vi "RCM Filter String MHLC.vi"(8 "error in (no error)":errorcluster, 10 "Data":variant, 11 "Message Log in":refnum<class "Message Log.lvclass">) -> (0 "error out":errorcluster, 3 "Message Log out":refnum<class "Message Log.lvclass">)   [LabVIEW 2017, in "Message Log.lvclass"]
doc: "Filter string on selected column"
uses:
  Message Log.lvclass
  rql_RCM Filter String.ctl
  Listbox Selection.ctl
  <vilib>/Utility/miscctls.llb/LVRowAndColumnTypeDef.ctl
  Message Log.lvclass/Message Log.ctl
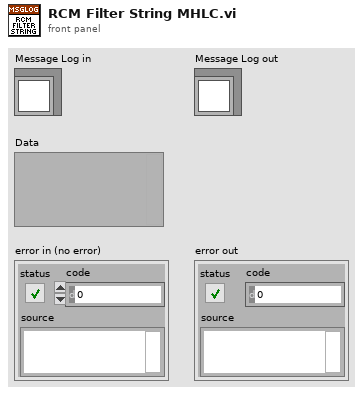
[diagram p1: front panel]
types:
  T1 = typedef "Message Log.lvclass/rql_RCM Filter String.ctl" = cluster{"RCM Listbox Data":T2}
  T2 = typedef "Message Log.lvclass/Listbox Selection.ctl" = cluster{"Cell Position":T3, "Row":string[]}
  T3 = typedef "LVRowAndColumnTypeDef.ctl" = cluster{"Row":i32, "Column":i32}
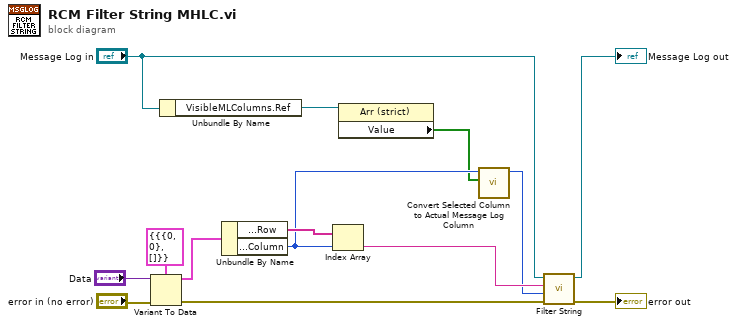
[diagram p0: block diagram]
diagram:
  n1 = Variant To Data(error in="error in (no error)", type=T1 {"RCM Listbox Data"={"Cell Position"={"Row"=0, "Column"=0}, "Row"=[]}} ("Data"), Variant="Data") -> (data=w13:T1, error out=w4:errorcluster)
  n2 = Unbundle By Name("Message Log in") -> ("VisibleMLColumns.Ref"=w8:refnum<vi>)
  n3 = Unbundle By Name(w13) -> ("RCM Listbox Data.Row"=w10:string[], "RCM Listbox Data.Cell Position.Column"=w9:i32)
  n4 = Index Array(array=w10, index=w9) -> (element=w6:string)
  n5 = property class="Arr (strict)"(reference=w8) -> ("Value"=w7:bool[])  [unwired: 1 in, 2 out]
  n6 = call "Convert Selected Column to Actual Message Log Column.vi"("Visible ML Columns"=w7, "Selected Column"=w9) -> ("Actual Column"=w5:i32)  [unwired: 9 in]
  n7 = call "Filter String.vi"("error in (no error)"=w4, "Actual Column"=w5, "Filter String"=w6, "Message Log in"="Message Log in") -> ("error out"=→"error out":errorcluster, "Message Log out"=→"Message Log out":refnum<class "Message Log.lvclass">)  [unwired: 6 in]
